vi "Read Registered Sinks.vi"(0 "Event Source in":refnum<class "Event Source.lvclass">, 5 "error in (no error)":errorcluster) -> (14 "Event Source out":refnum<class "Event Source.lvclass">, 19 "error out":errorcluster)   [LabVIEW 2016, in "Event Source.lvlib" / "Event Source.lvclass"]
doc: "Allows to set the Sink behaviour by setting the following flags\n\n\"Exclude From Broadcast\"\nmessage originating form another sink will not be broadcasted to the sink being cosidered\n\"Paused\"\nThe sink will not send events and will not receive them anymore\n\"Receive only\"\nThe sing will receive events but not sany any"
uses:
  Event Source.lvclass
  Event Source.lvclass/Event Source.ctl
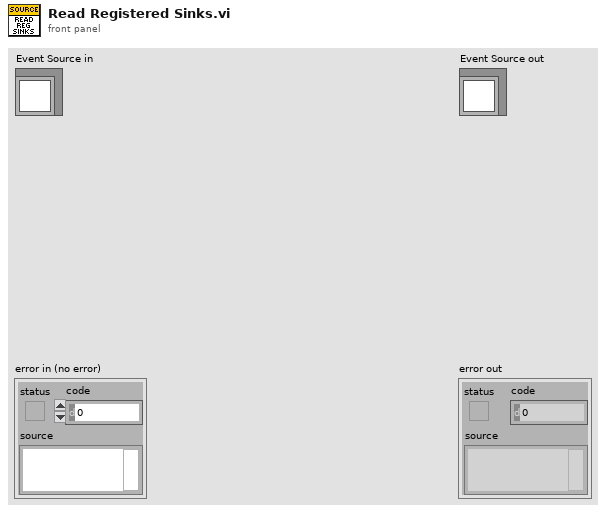
[diagram p1: front panel]
types:
  T1 = typedef "Event Source.lvlib/Event Source.lvclass/Registered Sinks Event Ref.ctl" = refnum<user-event>
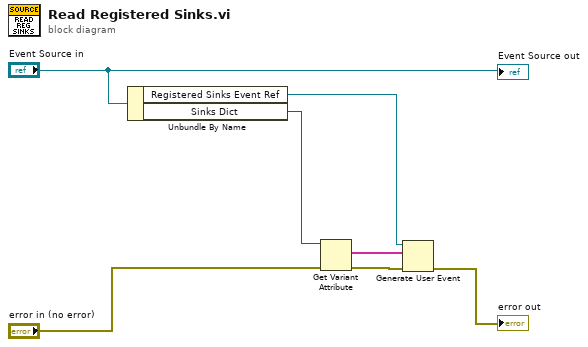
[diagram p0: block diagram]
diagram:
  n1 = Unbundle By Name("Event Source in") -> ("Registered Sinks Event Ref"=w2:T1, "Sinks Dict"=w7:variant)
  n2 = Get Variant Attribute(Variant=w7, error in="error in (no error)") -> (names=w1:string[], error out=w4:errorcluster)  [unwired: 2 in, 2 out]
  n3 = Generate User Event(user event=w2, event data cluster=w1, error in=w4) -> (error out=→"error out":errorcluster)  [unwired: 1 in, 1 out]
  "Event Source out" <- "Event Source in"
